vi "TLPM Close2.vi"(8 "error in (no error)":errorcluster, 11 "instrument handle":refnum<visa-resource-name>) -> (0 "error out":errorcluster)   [LabVIEW 2023, in "Thorlabs Power Meter.lvlib"]
doc: "This VI closes the instrument driver session.\n\nNote: The instrument must be reinitialized to use it again."
uses:
  Thorlabs Power Meter.lvlib
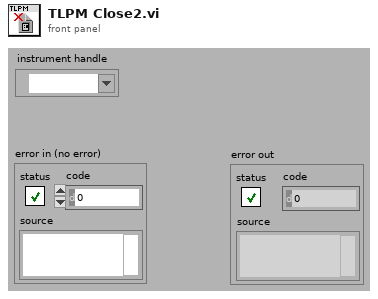
[diagram p1: front panel]
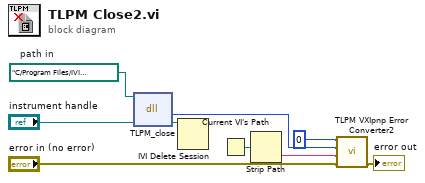
[diagram p0: block diagram]
diagram:
  w1 = path "C:/Program Files/IVI Foundation/VISA/Win64/Bin/TLPM_64.dll"  # path in
  n1 = dll-call lib="TLPM_64.dll" fn="TLPM_close"(path in=w1, "instrument handle"="instrument handle") -> ("status"=w3:i32)  [unwired: 3 in, 2 out]
  n2 = IVI Delete Session(11:"instrument handle") -> ()
  n3 = Current VI's Path() -> (path=w8:path)
  n4 = Strip Path(path=w8) -> (name=w4:string)  [unwired: 1 out]
  n5 = call "TLPM VXIpnp Error Converter2.vi"("error in (no error)"="error in (no error)", "Name Of VI (\"\")"=w4, "CVI Error Code (0)"=w3, "instrument handle"=i8 0) -> ("error out"=→"error out":errorcluster)  [unwired: 6 in, 1 out]
